vi "oa_Create Time Indice.vi"(0 "scaled signal [EU]":waveform(dbl)={"t0"=timestamp(0 s since 1904-01-01), "dt"=0.0, "Y"=[]}, 1 "reset? (True)":bool, 7 "steps":cluster{"start":dbl, "end":dbl, "step":dbl} {"step" format="%.2f"; "end" format="%.2f"; "start" format="%.2f"}, 11 "error in (no error)":errorcluster, 12 "step found?(F)":bool) -> (3 "signal processed":dbl format="%.2f", 4 "scaled signal [EU] dup":waveform(dbl), 6 "time indices":dbl[](array[numeric]) format="%.2f", 8 "scale":cluster{"offset":dbl, "multiplier":dbl} {"multiplier" format="%.2f"; "offset" format="%.2f"}, 10 "finished?":bool, 15 "error out":errorcluster)   [LabVIEW 2017]
uses:
  <vilib>/Waveform/WDTOps.llb/WDT Waveform Duration DBL.vi
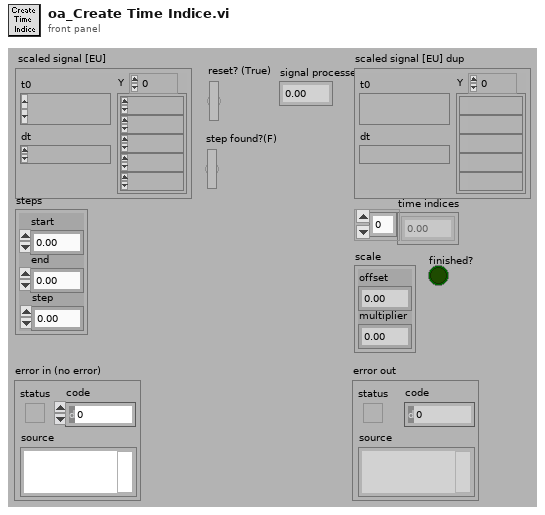
[diagram p1: front panel]
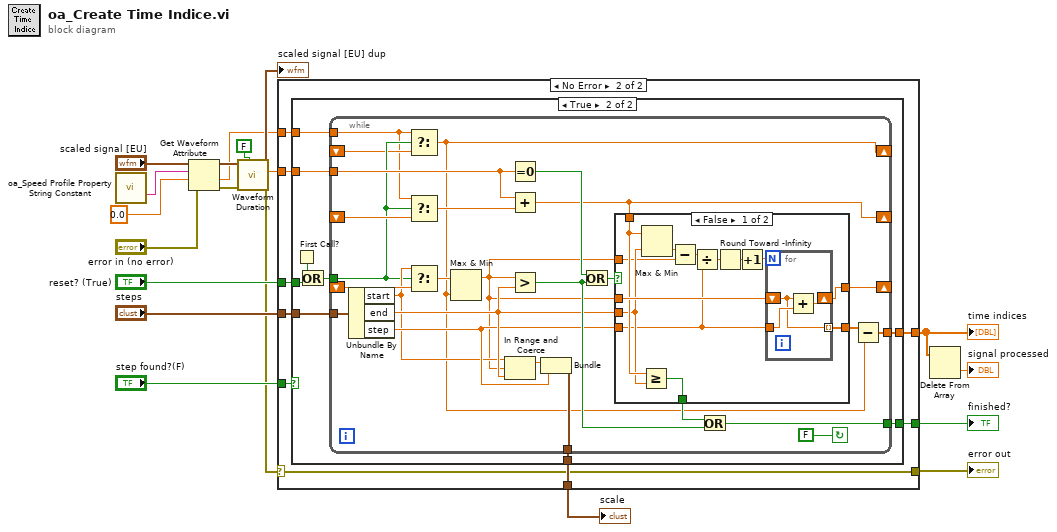
[diagram p0: block diagram]
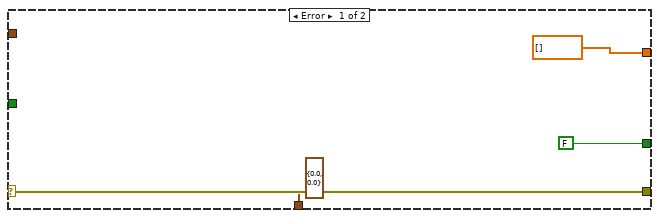
[diagram p2: hidden frame]
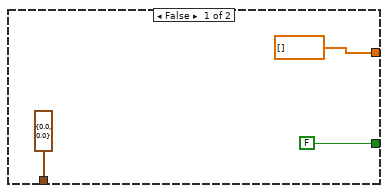
[diagram p3: hidden frame]
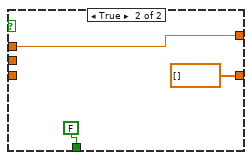
[diagram p4: hidden frame]
diagram:
  n1 = call <vilib>:"oa_Speed Profile Property String Constant.vi"() -> ("elapsed time"=w8:string)  [unwired: 12 in, 3 out]
  n2 = Get Waveform Attribute(4:"error in (no error)", 5:0.0, 6:w8, 7:"scaled signal [EU]") -> (0:w5:errorcluster, 1:w2:dbl, 3:w3:waveform(dbl))  [unwired: 1 out]
  n3 = call-poly <vilib>:"Waveform Duration.vi"("open interval? (T)"=FALSE, "error in (no error)"=w5, "waveform in"=w3) -> ("error out"=w11:errorcluster, "duration"=w10:dbl, "waveform out"=→"scaled signal [EU] dup":waveform(dbl))  [unwired: 6 in]
  n4 = case shown="No Error" w11 {
    selector: w11 -> [w23 w26]
    tunnel: "steps" -> [_ w32]
    tunnel: [FALSE w31] -> w18
    tunnel: "reset? (True)" -> [_ w30]
    tunnel: w10 -> [_ w29]
    tunnel: [cluster{"start":dbl, "step":dbl} {"start"=0.0, "step"=0.0} w28] -> w16
    tunnel: [dbl[] [] w27] -> w1
    tunnel: [w23 w26] -> w15
    tunnel: "step found?(F)" -> [_ w25]
    tunnel: w2 -> [_ w24]
    frame Error {
    }
    frame No Error {
      n5 = case shown="True" w25 {
        tunnel: w32 -> [_ w44]
        tunnel: [FALSE w43] -> w31
        tunnel: w30 -> [_ w42]
        tunnel: w29 -> [_ w39]
        tunnel: [cluster{"start":dbl, "step":dbl} {"start"=0.0, "step"=0.0} w38] -> w28
        tunnel: [dbl[] [] w37] -> w27
        tunnel: w24 -> [_ w36]
        frame False {
        }
        frame True {
          n6 = First Call?() -> (First Call?: T/F=w40:bool)
          n7 = Or(x=w40, y=w42) -> (x .or. y?=w41:bool)
          n8 = while {
            shift-right: [w56] -> _
            shift-left: _ -> [w69]
            tunnel: w41 -> [w50]
            tunnel: w39 -> [w65]
            tunnel: w44 -> [w67]
            shift-right: [w57] -> _
            shift-left: _ -> [w66]
            tunnel: [w60] -> w43
            tunnel: [w58] -> w38
            tunnel: [w47] -> w37
            tunnel: w36 -> [w45]
            shift-right: [w48] -> _
            shift-left: _ -> [w49]
            stop <- FALSE continue-if-true
            n9 = Unbundle By Name(w67) -> ("start"=w53:dbl, "end"=w59:dbl, "step"=w55:dbl)
            n10 = Select(t=w45, s=w50, f=w49) -> (s? t:f=w48:dbl)
            n11 = Select(t=w45, s=w50, f=w69) -> (s? t:f=w68:dbl)
            n12 = Select(t=w53, s=w50, f=w66) -> (s? t:f=w52:dbl)
            n13 = Max & Min(x=w52, y=w48) -> (max(x,y)=w51:dbl)  [unwired: 1 out]
            n14 = In Range and Coerce(upper limit=w53, x=w51, lower limit=w59) -> (coerced(x)=w54:dbl)  [unwired: 1 out]
            n15 = Equal To 0?(x=w65) -> (x = 0?=w64:bool)
            n16 = Add(x=w65, y=w68) -> (x+y=w56:dbl)
            n17 = Greater?(x=w51, y=w59) -> (0:w61:bool)
            n18 = Bundle("start"=w54, "step"=w55) -> (w58:cluster{"start":dbl, "step":dbl})  [unwired: 1 in]
            n19 = Or(x=w64, y=w61) -> (x .or. y?=w63:bool)
            n20 = case shown="False" w63 {
              tunnel: w59 -> [w78 _]
              tunnel: w51 -> [w82 w88]
              tunnel: w56 -> [w79 _]
              tunnel: w55 -> [w74 _]
              tunnel: [w80 FALSE] -> w62
              tunnel: [w77 w88] -> w57
              tunnel: [w81 dbl[] []] -> w46
              tunnel: w51 -> [w76 _]
              frame False {
                n21 = Greater Or Equal?(x=w79, y=w78) -> (x >= y?=w80:bool)
                n22 = Max & Min(x=w79, y=w78) -> (min(x,y)=w83:dbl)  [unwired: 1 out]
                n23 = Subtract(x=w83, y=w76) -> (x-y=w75:dbl)
                n24 = Divide(x=w75, y=w74) -> (x/y=w73:dbl)
                n25 = Round Toward -Infinity(1:w73) -> (0:w71:dbl)
                n26 = Increment(x=w71) -> (x+1=w72:dbl)
                n27 = for {
                  N: w72 -> [_]
                  tunnel: w74 -> [w86]
                  shift-right: [w85] -> w77
                  shift-left: w82 -> [w84]
                  tunnel: [w84] -> w81 mode=indexing
                  n28 = Add(x=w84, y=w86) -> (x+y=w85:dbl)
                }
              }
              frame True {
              }
            }
            n29 = Or(x=w62, y=w61) -> (x .or. y?=w60:bool)
            n30 = Subtract(x=w46, y=w48) -> (x-y=w47:dbl[])
          }
        }
      }
    }
  }
  "scale" <- w16
  "time indices" <- w1
  "finished?" <- w18
  "error out" <- w15
  n31 = Delete From Array(array=w1) -> (deleted portion=→"signal processed":dbl)  [unwired: 2 in, 1 out]
